vi "sendHeader.vi"(8 "error in (no error)":errorcluster, 10 "MessageHeader":T1, 11 "M1M3SAL in":refnum<class "M1M3SAL.lvclass">) -> (0 "error out":errorcluster, 3 "M1M3SAL out":refnum<class "M1M3SAL.lvclass">)   [LabVIEW 2016, in "M1M3SupportCommunicator.lvlib" / "M1M3SAL.lvclass"]
uses:
  M1M3SAL.lvclass
  DataTypes/MessageHeader.ctl
  DataTypes/MessageTypes.ctl
  DataTypes/MessageTopics.ctl
  Common_RT_Utilities/U8ArrayBuilderAutoIndexing/U8ArrayBuilderAutoIndexing.lvclass
  M1M3SupportCommunicator.lvlib
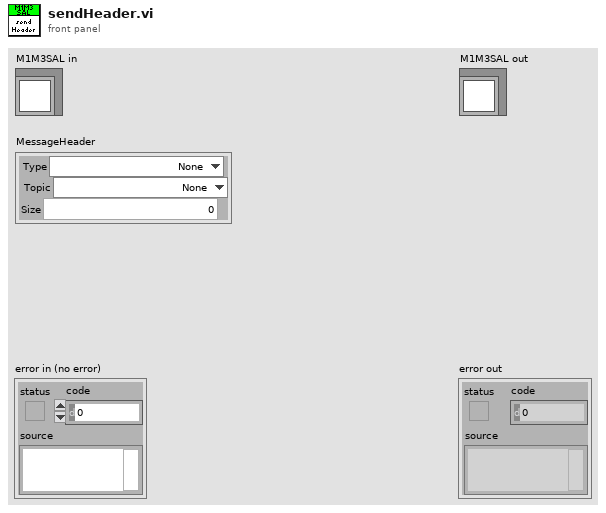
[diagram p1: front panel]
types:
  T1 = typedef "M1M3SupportCommunicator.lvlib/MessageHeader.ctl" = cluster{"Type":T2, "Topic":T3, "Size":i32}
  T2 = typedef "M1M3SupportCommunicator.lvlib/MessageTypes.ctl" = enum8{"None", "PutSample", "GetNextSample", "LogEvent", "GetEvent", "IssueCommand", "CommandId", "WaitForCompletion", "AcceptCommand", "AckCommand"}
  T3 = typedef "M1M3SupportCommunicator.lvlib/MessageTopics.ctl" = enum8{"None", "Start", "Enable", "Disable", "Standby", "AppliedSettingsMatchStart", "ErrorCode", "SettingVersions", "SummaryState", "DetailedState", "Exit"}
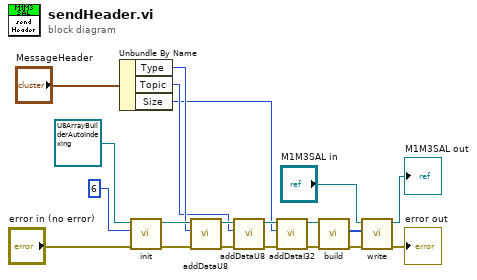
[diagram p0: block diagram]
diagram:
  n1 = Unbundle By Name("MessageHeader") -> ("Type"=w13:T2, "Topic"=w12:T3, "Size"=w11:i32)
  n2 = call "init.vi"("error in (no error)"="error in (no error)", "Size"=6, "U8ArrayBuilderAutoIndexing in"=refnum<class "U8ArrayBuilderAutoIndexing.lvclass"> refnum ("RTUtilities.lvlib:U8ArrayBuilderAutoIndexing.lvclass")) -> ("error out"=w10:errorcluster, "U8ArrayBuilderAutoIndexing out"=w17:refnum<class "U8ArrayBuilderAutoIndexing.lvclass">)  [unwired: 7 in]
  n3 = call "addDataU8.vi"("error in (no error)"=w10, "Data"=w13, "U8ArrayBuilderAutoIndexing in"=w17) -> ("error out"=w9:errorcluster, "U8ArrayBuilderAutoIndexing out"=w16:refnum<class "U8ArrayBuilderAutoIndexing.lvclass">)  [unwired: 7 in]
  n4 = call "addDataU8.vi"("error in (no error)"=w9, "Data"=w12, "U8ArrayBuilderAutoIndexing in"=w16) -> ("error out"=w8:errorcluster, "U8ArrayBuilderAutoIndexing out"=w15:refnum<class "U8ArrayBuilderAutoIndexing.lvclass">)  [unwired: 7 in]
  n5 = call "addDataI32.vi"("error in (no error)"=w8, "Data"=w11, "U8ArrayBuilderAutoIndexing in"=w15) -> ("error out"=w7:errorcluster, "U8ArrayBuilderAutoIndexing out"=w14:refnum<class "U8ArrayBuilderAutoIndexing.lvclass">)  [unwired: 7 in]
  n6 = call "build.vi"("error in (no error)"=w7, "U8ArrayBuilderAutoIndexing in"=w14) -> ("error out"=w5:errorcluster, "Array"=w6:u8[])  [unwired: 7 in, 1 out]
  n7 = call "write.vi"("error in (no error)"=w5, "Data"=w6, "M1M3SAL in"="M1M3SAL in") -> ("error out"=→"error out":errorcluster, "M1M3SAL out"=→"M1M3SAL out":refnum<class "M1M3SAL.lvclass">)  [unwired: 7 in]
